vi "Initialize Serial.vi"(7 "timeout, ms (1000)":u32=1000, 8 "error in (no error)":errorcluster, 10 "baud rate (115200)":u32(ring)=115200 items=["9600"=9600, "19200"=19200, "38400"=38400, "57600"=57600, "115200"=115200], 11 "port":refnum<visa-resource-name>) -> (0 "error out":errorcluster, 3 "VGC out":refnum<class "PL Inficon VGC.lvclass">)   [LabVIEW 2015, in "PL Inficon VGC.lvclass"]
doc: "Initializes connection to device using specified settings."
uses:
  PL Inficon VGC.lvclass
  PL Inficon VGC.lvclass/PL Inficon VGC.ctl
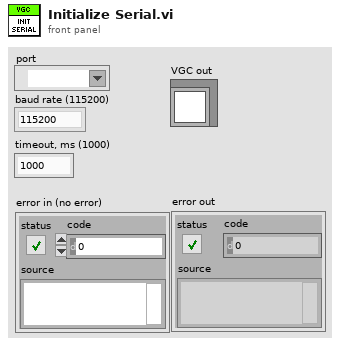
[diagram p1: front panel]
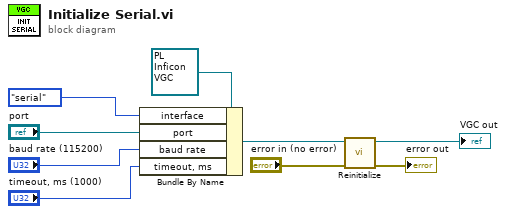
[diagram p0: block diagram]
diagram:
  n1 = Bundle By Name(cluster=refnum<class "PL Inficon VGC.lvclass"> refnum, "interface"=enum16{"serial", "network"}."serial", "port"="port", "baud rate"="baud rate (115200)", "timeout, ms"="timeout, ms (1000)") -> (w9:refnum<class "PL Inficon VGC.lvclass">)
  n2 = call "Reinitialize.vi"("error in (no error)"="error in (no error)", "VGC in"=w9) -> ("error out"=→"error out":errorcluster, "VGC out"=→"VGC out":refnum<class "PL Inficon VGC.lvclass">)  [unwired: 8 in]
